vi "AuMT8852B Link Timeout.vi"(5 "Timeout (10 s)":i32=10, 7 "Set/Get (Set)":enum16{"Set", "Get"}(ring), 8 "error in (no error)":errorcluster, 11 "VISA session":refnum<visa-resource-name>) -> (0 "error out":errorcluster, 2 "error code":i32, 3 "VISA session out":refnum<visa-resource-name>, 4 "Timeout out":i32=10)   [LabVIEW 2017]
doc: "Anritsu MT8852B Bluetooth Tester\n\nNumber of seconds the tester will wait after losing a connection before abandoning the link.\n\nINPUTS\nSet/Get - whether the value is being sent to or retrieved from the instrument.\nTimeout - seconds to wait (1-40).\n\nOUTPUTS\nTimeout out - timeout value currently being used."
uses:
  <instrlib>/aumt8852B/General/Utilities/MT8850 Attribute ID.ctl
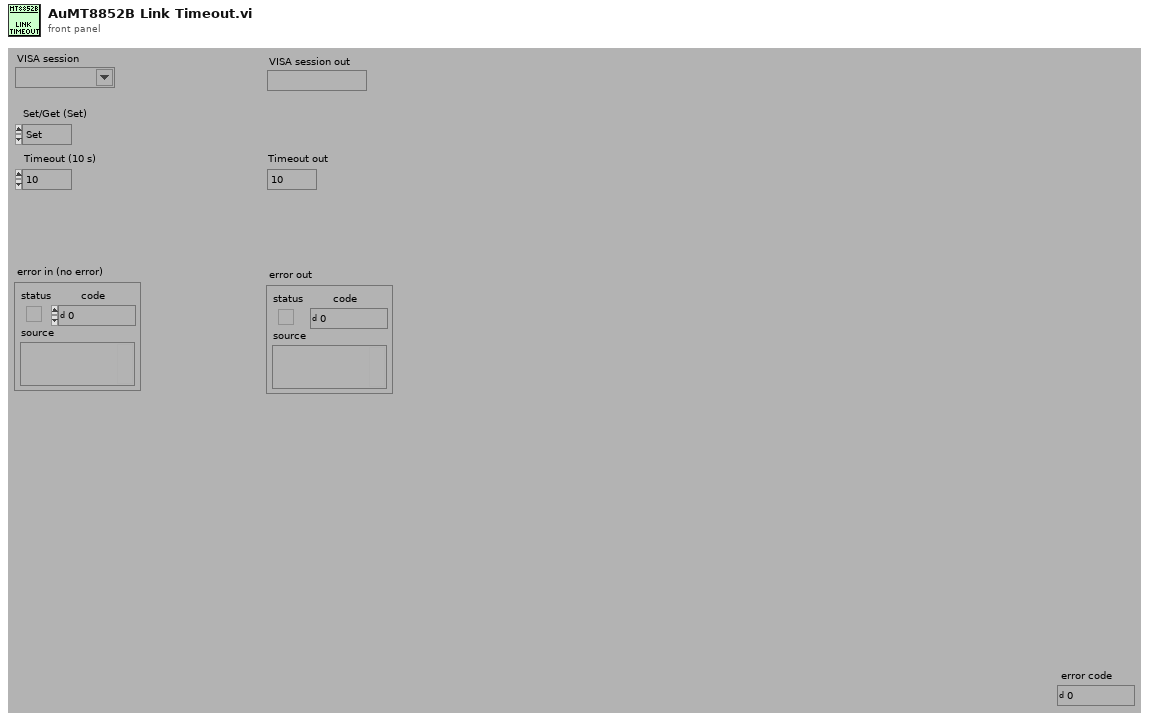
[diagram p1: front panel]
types:
  T1 = typedef "MT8850 Attribute ID.ctl" = enum16{"Operation mode", "Selected script", "EUT address source", "EUT Address", "EUT HCI RS232 Baud Rate", "Tester GPIB Address", "Tester RS232 Baud Rate", "Tester Bluetooth Address", "Tester Contrast", "Tester Key Click On", "Tester Modulation Index", "Tester Poll-Null Mode", "Tester Power Range", "Tester RS232 Mode", "Beep on Illegal Entry", "Display User Text", "User Text", "Calibration TX Modulation DAC", "Calibration RX Channel", "Calibration TX Channel", "Calibration TX Power", "Calibration Use TX Table", "Inquiry Request User-friendly Name", "Inquiry Number of Responses", "Inquiry Timeout", "Script Frequency Display", "Script Loop Count", "Script Loop Continuously", "Script Loop Stop on Fail", "Link timeout", "Page timeout", "Filter bandwidth", "SCO air code", "SCO bit position", "SCO input code", "SCO input data", "SCO input sample size", "SCO loopback mode", "SCO packet type", "SCO tone generator", "Tester page scan repetition mode", "Tester follow test mode", "Tester authentication state", "Tester authentication pin code", "Tester authentication pin length"}
  T2 = typedef "Attribute Status.ctl" = enum16{"No I/O needed", "I/O needed"}
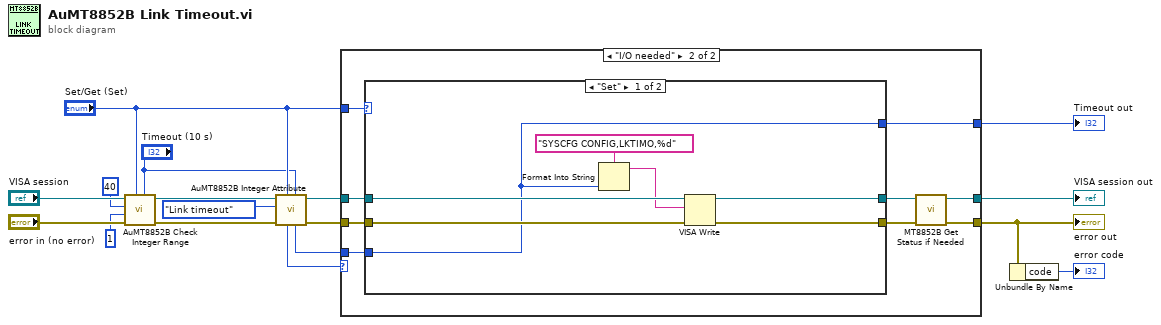
[diagram p0: block diagram]
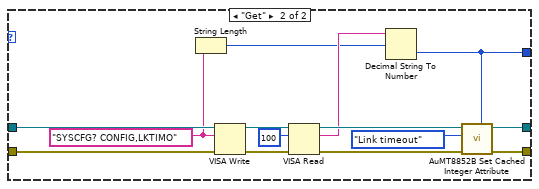
[diagram p3: hidden frame]
diagram:
  n1 = call <instrlib>:"AuMT8852B Check Integer Range.vi"("Value (0)"="Timeout (10 s)", "Set/Get (Set)"="Set/Get (Set)", "error in (no error)"="error in (no error)", "Lower limit (-1)"=1, "Upper limit (1)"=40, "VISA session"="VISA session") -> ("error out"=w7:errorcluster, "VISA session out"=w8:refnum<visa-resource-name>)  [unwired: 4 in]
  n2 = call <instrlib>:"AuMT8852B Integer Attribute.vi"("Value (0)"="Timeout (10 s)", "Set/Get (Set)"="Set/Get (Set)", "error in (no error)"=w7, "Attribute ID"=MT8850_Attribute_ID."Link timeout", "VISA session"=w8) -> ("error out"=w13:errorcluster, "VISA session out"=w14:refnum<visa-resource-name>, "Value out"=w16:i32, "Status"=w12:T2)  [unwired: 3 in]
  n3 = case shown="\"I/O needed\"" w12 {
    tunnel: "Set/Get (Set)" -> [_ w29]
    tunnel: w16 -> [w20 w28]
    tunnel: [w18 w21] -> w1
    tunnel: [w19 w22] -> w15
    tunnel: w14 -> [w19 w27]
    tunnel: w13 -> [w18 w26]
    tunnel: [w20 w25] -> w11
    frame "No I/O needed", Default {
    }
    frame "I/O needed" {
      n4 = case shown="\"Set\"" w29 {
        tunnel: [w33 w42] -> w23
        tunnel: w28 -> [w30 _]
        tunnel: [w34 w43] -> w24
        tunnel: w27 -> [w36 w50]
        tunnel: w26 -> [w35 w49]
        tunnel: [w30 w39] -> w25
        frame "Set" {
          n5 = Format Into String(format string="SYSCFG CONFIG,LKTIMO,%d" ("Format String"), w30) -> (resulting string=w31:string)  [unwired: 2 in, 1 out]
          n6 = VISA Write(VISA resource name=w36, write buffer=w31, error in (no error)=w35) -> (VISA resource name out=w34:refnum<visa-resource-name>, error out=w33:errorcluster)  [unwired: 1 out]
        }
        frame "Get" {
          w38 = "SYSCFG? CONFIG,LKTIMO" ("write buffer (\"\")")
          n7 = String Length(string=w38) -> (length=w37:i32)
          n8 = VISA Write(VISA resource name=w50, write buffer=w38, error in (no error)=w49) -> (VISA resource name out=w48:refnum<visa-resource-name>, error out=w46:errorcluster)  [unwired: 1 out]
          n9 = VISA Read(VISA resource name=w48, byte count=u32 100 ("byte count (0)"), error in (no error)=w46) -> (VISA resource name out=w45:refnum<visa-resource-name>, read buffer=w40:string, error out=w44:errorcluster)  [unwired: 1 out]
          n10 = Decimal String To Number(string=w40, offset=w37) -> (number=w39:i32)  [unwired: 1 in, 1 out]
          n11 = call <instrlib>:"AuMT8852B Set Cached Integer Attribute.vi"("Value (0)"=w39, "error in (no error)"=w44, "Attribute ID"=MT8850_Attribute_ID."Link timeout", "VISA session"=w45) -> ("error out"=w42:errorcluster, "VISA session out"=w43:refnum<visa-resource-name>)  [unwired: 6 in]
        }
      }
      n12 = call <instrlib>:"MT8852B Get Status if Needed.vi"("error in (no error)"=w23, "VISA session"=w24) -> ("error out"=w21:errorcluster, "VISA session out"=w22:refnum<visa-resource-name>)  [unwired: 8 in]
    }
  }
  "error out" <- w1
  "VISA session out" <- w15
  "Timeout out" <- w11
  n13 = Unbundle By Name(w1) -> ("code"=→"error code":i32)
